vi "key.vi"(10 "node ref in":refnum<data-value>, 11 "adstar in":refnum<class "NI_Robotics_AnytimeDStar.lvclass">) -> (1 "key out":cluster{"(g or v) + h":dbl, "g or v":dbl}, 2 "node ref out":refnum<data-value>, 3 "adstar out":refnum<class "NI_Robotics_AnytimeDStar.lvclass">)   [LabVIEW 2017, in "NI_Robotics_AnytimeDStar.lvclass"]
uses:
  <vilib>/robotics/Navigation/Anytime D Star/NI_Robotics_AnytimeDStar.lvclass
  <vilib>/robotics/Navigation/shared/MapNode/AbstractDstarNode/NI_Robotics_AbstractDstarNode.lvclass
  c:/Program Files (x86)/National Instruments/LabVIEW 2017/vi.lib/robotics/Navigation/shared/MapNode/AbstractMapNode/NI_Robotics_AbstractMapNode.lvclass
  <vilib>/robotics/Navigation/Anytime D Star/NI_Robotics_AnytimeDStar.lvclass/NI_Robotics_AnytimeDStar.ctl
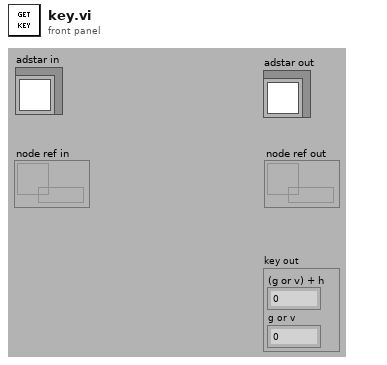
[diagram p1: front panel]
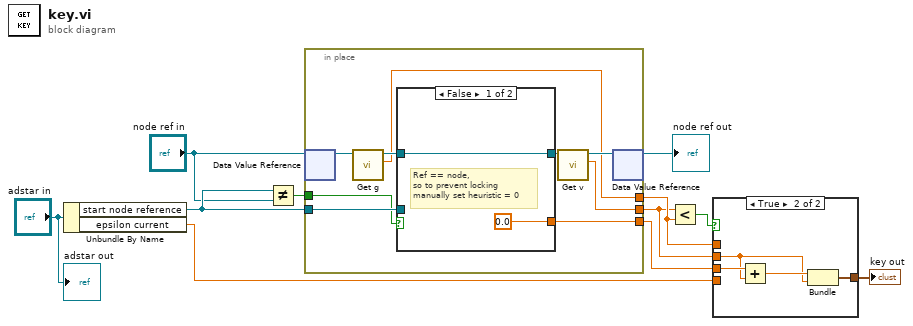
[diagram p0: block diagram]
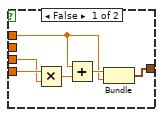
[diagram p2: hidden frame]
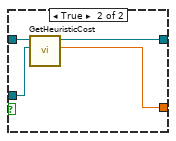
[diagram p3: hidden frame]
diagram:
  n1 = Unbundle By Name("adstar in") -> ("start node reference"=w2:refnum<data-value>, "epsilon current"=w4:dbl)
  n2 = Not Equal?(x=w2, y="node ref in") -> (x != y?=w3:bool)
  n3 = in-place {
    in-place-border: w2 -> [w16]
    in-place-border: [w15] -> w6
    in-place-border: [w14] -> w9
    in-place-border: [w13] -> w7
    in-place-border: w3 -> [w12]
    n4 = in-place-dvr #1("node ref in") -> (w19:refnum<class "NI_Robotics_AbstractDstarNode.lvclass">)  [unwired: 1 out]
    n5 = call <vilib>:"Get g.vi"("AbstractDstarNode in"=w19) -> ("g"=w13:dbl, "AbstractDstarNode out"=w18:refnum<class "NI_Robotics_AbstractDstarNode.lvclass">)  [unwired: 9 in]
    n6 = case shown="False" w12 {
      tunnel: [0.0 ("Hueristic Cost") w26] -> w14
      tunnel: w18 -> [w22 w25]
      tunnel: [w22 w24] -> w17
      tunnel: w16 -> [_ w23]
      frame False {
        # "Ref == node,\nso to prevent locking\nmanually set heuristic = 0"
      }
      frame True {
        n7 = call-dynamic "GetHeuristicCost.vi"("Goal NodeReference"=w23, "AbstractAstarNode in"=w25) -> ("hueristic cost"=w26:dbl, "AbstractAstarNode out"=w24:refnum<class "NI_Robotics_AbstractDstarNode.lvclass">)  [unwired: 7 in, 1 out]
      }
    }
    n8 = call <vilib>:"Get v.vi"("AbstractDstarNode in"=w17) -> ("v"=w15:dbl, "AbstractDstarNode out"=w20:refnum<class "NI_Robotics_AbstractDstarNode.lvclass">)  [unwired: 9 in]
    n9 = in-place-dvr #1(w20) -> (→"node ref out":refnum<data-value>)  [unwired: 1 out]
  }
  n10 = Less?(x=w6, y=w7) -> (x < y?=w5:bool)
  n11 = case shown="True" w5 {
    tunnel: [w27 w36] -> w8
    tunnel: w9 -> [w28 w34]
    tunnel: w6 -> [_ w33]
    tunnel: w7 -> [w30 _]
    tunnel: w4 -> [w29 _]
    frame False {
      n12 = Multiply(x=w29, y=w28) -> (x*y=w31:dbl)
      n13 = Add(x=w30, y=w31) -> (x+y=w32:dbl)
      n14 = Bundle(w32, "g"=w30) -> (w27:cluster{dbl, "g":dbl})  [unwired: 1 in]
    }
    frame True {
      n15 = Add(x=w34, y=w33) -> (x+y=w35:dbl)
      n16 = Bundle(w35, "v"=w33) -> (w36:cluster{dbl, "v":dbl})  [unwired: 1 in]
    }
  }
  "key out" <- w8
  "adstar out" <- "adstar in"
